vi "Measure-Power_PM.vi"(8 "error in (no error)":errorcluster {"code" format="%.0x"}, 9 "Numeric":i32, 10 "Sensor":string, 11 "instrument handle":refnum<visa-resource-name>) -> (0 "error out":errorcluster, 2 "Power":dbl, 3 "instrument handle out":refnum<visa-resource-name>)   [LabVIEW 2018]
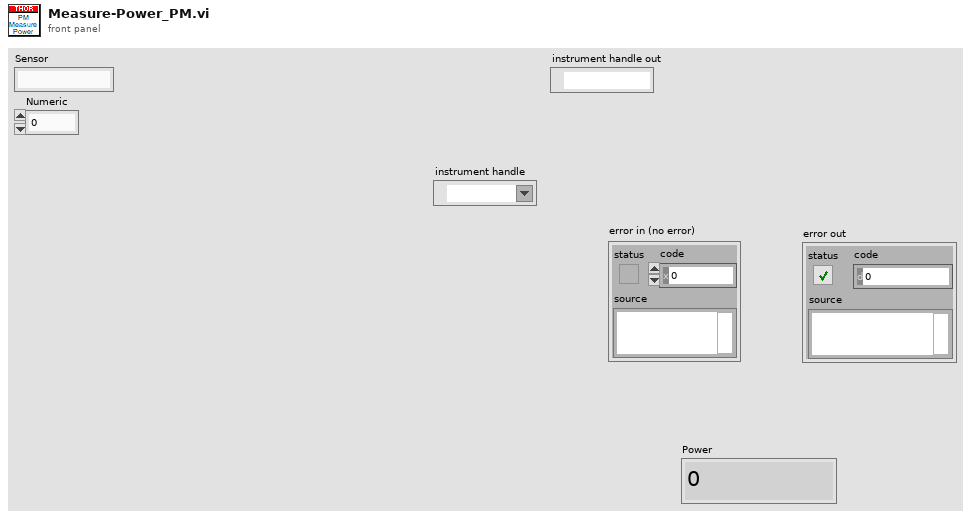
[diagram p1: front panel]
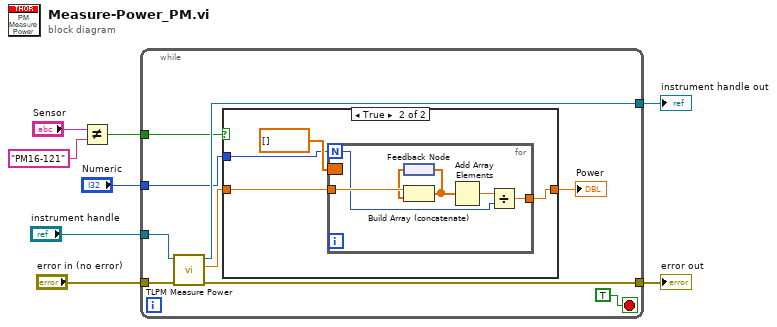
[diagram p0: block diagram]
diagram:
  n1 = Not Equal?(x="Sensor", y="PM16-121") -> (x != y?=w3:bool)
  n2 = while {
    tunnel: "instrument handle" -> [w16]
    tunnel: [w14] -> w6
    tunnel: "error in (no error)" -> [w15]
    tunnel: [w13] -> w5
    tunnel: w3 -> [w11]
    tunnel: "Numeric" -> [w10]
    stop <- TRUE stop-if-true
    n3 = call "TLPM Measure Power.vi"("error in (no error)"=w15, "instrument handle"=w16) -> ("error out"=w13:errorcluster, "Power"=w12:dbl, "instrument handle out"=w14:refnum<visa-resource-name>)  [unwired: 7 in]
    n4 = case shown="True" w11 {
      tunnel: w12 -> [w18 w22]
      tunnel: w10 -> [_ w20]
      tunnel: [w18 w19] -> w9
      frame False {
      }
      frame True {
        n5 = for {
          N: w20 -> [w25]
          tunnel: w22 -> [w28]
          border: dbl[] [] -> [_]
          tunnel: [w23] -> w19
          n6 = feedback #1() -> (w27:dbl[])
          n7 = Build Array (concatenate)(w28, w27) -> (w24:dbl[])
          n8 = feedback-in #1(w24) -> ()
          n9 = Add Array Elements(numeric array=w24) -> (sum=w26:dbl)
          n10 = Divide(x=w26, y=w25) -> (x/y=w23:dbl)
        }
      }
    }
    "Power" <- w9
  }
  "error out" <- w5
  "instrument handle out" <- w6
